vi "read_randoms.vi"() -> ()   [LabVIEW 2018]
panel:
  in  "file path (use dialog)":path
  in  "stop":bool
  in  "?":bool
  out "String":string
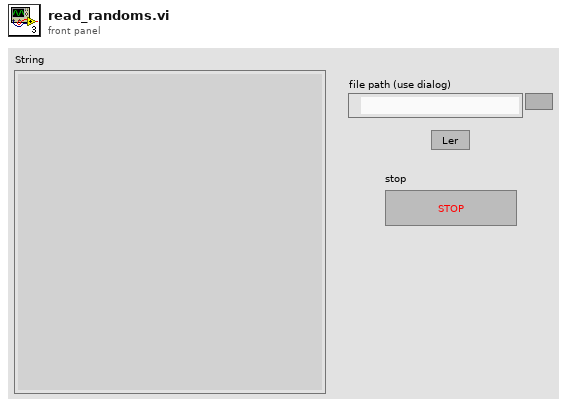
[diagram p1: front panel]
types:
  T1 = enum16{"open", "replace", "create", "open or create", "replace or create", "replace or create with confirmation"}
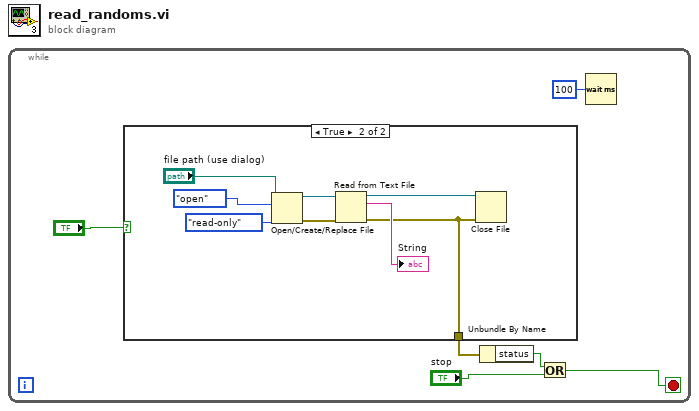
[diagram p0: block diagram]
diagram:
  n1 = while {
    stop <- w2 stop-if-true
    n2 = case shown="True" "?" {
      tunnel: [_ w7] -> w4
      frame False {
      }
      frame True {
        n3 = Open/Create/Replace File(file path (use dialog)="file path (use dialog)", operation (0:open)=T1."open", access (0:read/write)=enum16{"read/write", "read-only", "write-only"}."read-only") -> (refnum out=w11:refnum<file>, error out=w10:errorcluster)  [unwired: 3 in, 1 out]
        n4 = Read from Text File(file (use dialog)=w11, error in=w10) -> (refnum out=w9:refnum<file>, text=→"String":string, error out=w7:errorcluster)  [unwired: 2 in, 1 out]
        n5 = Close File(refnum=w9, error in=w7) -> ()  [unwired: 2 out]
      }
    }
    n6 = Unbundle By Name(w4) -> ("status"=w3:bool)
    n7 = Or(x=w3, y="stop") -> (x .or. y?=w2:bool)
    n8 = Wait (ms)(milliseconds to wait=u32 100) -> ()  [unwired: 1 out]
  }
